vi "2D Interpolated Table Lookup.vi"(0 "2d Input Table":dbl[][](array[numeric]), 1 "Input Row":dbl=20.0 format="%#_13g", 2 "Input Col":dbl=20.0 format="%#_13g", 5 "Max Row Range":dbl=100.0 format="%#_13g", 7 "Min Row Range":dbl format="%#_13g", 9 "Max Col Range":dbl=100.0 format="%#_13g", 11 "Min Col Range":dbl format="%#_13g") -> (4 "Output":dbl)   [LabVIEW 2013]
panel:
  out "columns":i32
  out "rows":i32
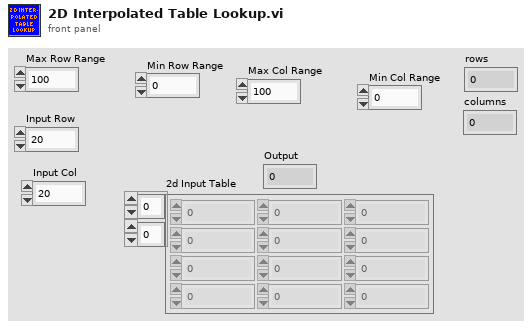
[diagram p1: front panel]
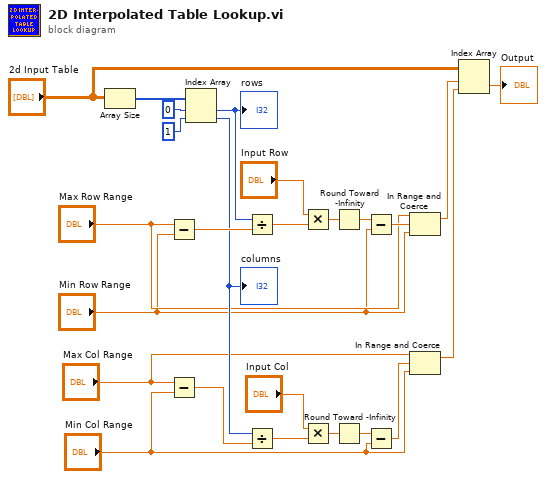
[diagram p0: block diagram]
diagram:
  n1 = Array Size(array="2d Input Table") -> (size(s)=w19:i32[])
  n2 = Subtract(x="Max Row Range", y="Min Row Range") -> (x-y=w20:dbl)
  n3 = Subtract(x="Max Col Range", y="Min Col Range") -> (x-y=w15:dbl)
  n4 = Index Array(array=w19, index #1=0 ("index"), index #2=1 ("index")) -> (element #1=w16:i32, element #2=w12:i32)
  "rows" <- w16
  "columns" <- w12
  n5 = Divide(x=w16, y=w20) -> (x/y=w22:dbl)
  n6 = Divide(x=w12, y=w15) -> (x/y=w13:dbl)
  n7 = Multiply(x="Input Row", y=w22) -> (x*y=w21:dbl)
  n8 = Multiply(x="Input Col", y=w13) -> (x*y=w14:dbl)
  n9 = Round Toward -Infinity(1:w21) -> (0:w9:dbl)
  n10 = Round Toward -Infinity(1:w14) -> (0:w10:dbl)
  n11 = Subtract(x=w9, y="Min Row Range") -> (x-y=w4:dbl)
  n12 = Subtract(x=w10, y="Min Col Range") -> (x-y=w8:dbl)
  n13 = In Range and Coerce(upper limit="Max Row Range", x=w4, lower limit="Min Row Range") -> (coerced(x)=w1:dbl)  [unwired: 1 out]
  n14 = In Range and Coerce(upper limit="Max Col Range", x=w8, lower limit="Min Col Range") -> (coerced(x)=w5:dbl)  [unwired: 1 out]
  n15 = Index Array(array="2d Input Table", index (row)=w1, index (col)=w5) -> (element=→"Output":dbl)
